vi "J1939 - Workspace Control.vi"() -> ()   [LabVIEW 2023, in "J1939 Workspace Object.lvlib"]
doc: "Sample numeric display item."
uses:
  J1939 Workspace Object.lvlib
  <vilib>/NI VeriStand/Display Template Support/DisplayTemplateSupport.llb/cluster_Screen Item Settings.ctl
  <vilib>/NI VeriStand/Display Template Support/DisplayTemplateSupport.llb/cluster_Graph Scale Settings.ctl
  <vilib>/NI VeriStand/Display Template Support/DisplayTemplateSupport.llb/cluster_Graph Plot Settings.ctl
  NationalInstruments.VeriStand.SystemStorage
  Workspace Shared/Types/UI.StateVariables.ctl
  <vilib>/NI VeriStand/Display Template Support/DisplayTemplateSupport.llb/enum_Display Template Handler Minimal To Widget Msg.ctl
  <vilib>/NI VeriStand/Execution/Workspace/SystemStateRegEventRef.ctl
  <vilib>/NI VeriStand/Execution/Workspace/Target State Info.ctl
  <vilib>/NI VeriStand/Execution/Workspace/Target State.ctl
  Workspace Shared/Types/Private Data.ctl
  <vilib>/NI/STM/TCP/TCP Connection Info.ctl
  <vilib>/NI/STM/SubVIs/MetaDataElement.ctl
  Addon/Addon Shared/Types/Error Cluster.ctl
  Addon/Addon Shared/Types/Error Types.ctl
  <vilib>/NI VeriStand/Display Template Support/DisplayTemplateSupport.llb/enum_Display Template Handler Minimal To Workspace.ctl
  <vilib>/NI VeriStand/Execution/Workspace/WorkspaceAPI.ctl
  <vilib>/NI VeriStand/Execution/Workspace/SystemStateEventRef.ctl
  Workspace Shared/Types/UI.Refs.ctl
  SubModules/CAN-Streaming-Support/Source/UIs/Workspace Shared/Types/Host Stream Queue Refs.ctl
  SubModules/CAN-Streaming-Support/Source/UIs/Workspace Shared/Types/Host Stream Queue Type.ctl
  SubModules/CAN-Streaming-Support/Source/UIs/Workspace Shared/Types/Host Stream Queue Command.ctl
  <vilib>/xnet/xnet.llb/XNET Frame CAN.ctl
  <vilib>/xnet/xnet.llb/XNET Frame Type CAN.ctl
  Addon/Support Libraries/J1939 Utilities/SubVIs/Convert CAN Arb ID to J1939 ID.vi
  <vilib>/NI VeriStand/Display Template Support/DisplayTemplateSupport.llb/sub_Display Template Handler Custom.vi
  Addon/Addon Shared/J1939 Addon Shared.lvlib
  <vilib>/NI/STM/NI STM.lvlib
  Workspace Shared/J1939 Workspace Shared.lvlib
  <vilib>/NI VeriStand/Execution/Workspace/NI_VS Workspace ExecutionAPI.lvlib
  Addon/Support Libraries/J1939 Utilities/J1939 Utilities.lvlib
  SubModules/CAN-Streaming-Support/Source/UIs/Workspace Shared/CAN Stream Support Workspace Shared.lvlib
  NationalInstruments.VeriStand.ClientAPI
panel:
  in  "Tab Control":enum32{"DTCs", "RQST", "RAW FRAME"}(tab)
  in  "Refresh Continuous":bool
  in  "Clear DTC":bool
  in  "Refresh DTCs":bool
  in  "DTCs":i32(listbox)
  in  "Addresses":string(tree)
  in  "Refresh Addresses":bool
  out "Response":string
  in  "Request":bool
  in  "PGN":u32 format="%.0x"
  in  "DA":u8(ring)
  in  "Clear Array":bool
  in  "RAW":bool
  out "Priority":u8 format="%02x"
  out "SA":u8 format="%02x"
  out "PGN":u32 format="%06x"
  in  "Identifier":u32 format="%08x"
  in  "Data":u8[](array[numeric])=[0, 0, 0, 0, 0, 0, 0, 0] format="%.0x"
  in  "Errors":bool
  out "Device":string
  in  "NIVS.Workspace Event":refnum<event-registration>
  in  "NIVS.Gateway IP Address":string
  in  "NIVS.System Definition Root":refnum<k24>
  in  "Item.Data":T1
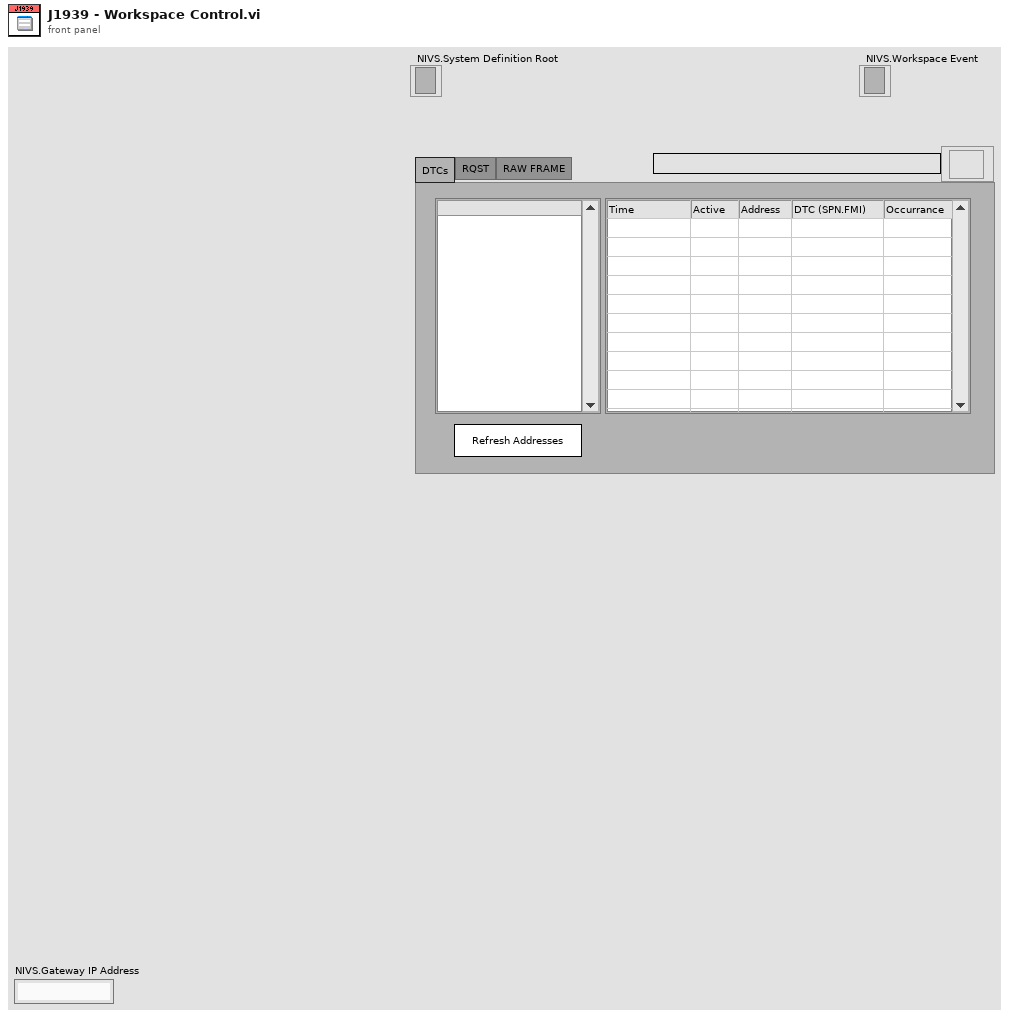
[diagram p1: front panel]
types:
  T1 = typedef "cluster_Screen Item Settings.ctl" = cluster{"Template VI":string, "Position X":i32, "Position Y":i32, "Custom":string, "Show Title Bar":bool, "ID":i32, "Always On Top":bool, "Allow Resize":bool, "Allow Minimize":bool, "Allow Close":bool, "Size to Screen":bool, "Screen.ID":i32, "State":enum16{"Normal", "New"}, "Title":string, "Window Bounds":cluster{"[0]":i16, "[1]":i16, "[2]":i16, "[3]":i16}, "Channel Ref":u64, "Unit":string, "Default Units?":bool, "Flash Limit?":bool, "Color 1":u32, "Color 2":u32, "Color 3":u32, "Color 4":u32, "Bck Color":u32, "Fore Color":u32, "Limit 1":dbl, "Limit 2":dbl, "Limit 3":dbl, "Limit 4":dbl, "Limit Mode 1":i32, "Limit Mode 2":i32, "Limit Mode 3":i32, "Limit Mode 4":i32, "Scale Precision":i32, "Scale Min":dbl, "Scale Max":dbl, "Format":i32, "Precision":i32, "Background Type":i32, "IDs":i32[], "Units":string[], "Labels":string[], "Scale Factor":dbl, "Scale Offset":dbl, "YScale Index":u32[], "XScale":T2, "YScales":T2[], "Plots":T3[], "Update Period":dbl, "History Length":dbl, "My.Ref":refnum<vi>, "Is Control?":bool, "Channel Paths":string[], "Custom Data":variant}
  T2 = typedef "cluster_Graph Scale Settings.ctl" = cluster{"Format":u8, "Precision":u8, "Fit":u8, "Label":string, "Use Default Label":bool, "Label Visible":bool, "Min":dbl, "Max":dbl}
  T3 = typedef "cluster_Graph Plot Settings.ctl" = cluster{"Bar Style":u8, "Fill To":i16, "Fill/PtColor":u32, "Line Style":u8, "Line Width":u8, "Color":u32, "Interp":u8, "Point Style":u8}
  T4 = typedef "J1939 Workspace Shared.lvlib/UI.StateVariables.ctl" = cluster{"NIVS.Gateway IP Address":string, "LaunchConfig.Ref":refnum<user-event>, "Events.Refs":cluster{"LaunchConfig":refnum<event-registration>, "SystemChange":T5, "NIVS.Workspace":refnum<event-registration>}, "State":T6, "TCP.Refs":T7, "Addresses.LUT":variant, "Errors.Q":refnum<queue>, "NIVS.SysDefRoot":refnum<k24>, "State.Notifier":refnum<user-event>, "NIVS.Workspace":T9, "DTCs.Refresh":bool, "NIVS.State.Refs":T10, "UI.Refs":T11, "Addon.Connected":bool, "DTCs.Timer":u32, "Mode.Tool?":bool, "Stream.Qs":T12, "NIVS.SysDef":path}
  T5 = typedef "NI_VS Workspace ExecutionAPI.lvlib/SystemStateRegEventRef.ctl" = refnum<event-registration>
  T6 = typedef "J1939 Workspace Shared.lvlib/Private Data.ctl" = cluster{"PGN":u32, "DA":u8, "CD Path":string, "CD IP":string}
  T7 = typedef "NI STM.lvlib/TCP Connection Info.ctl" = cluster{"connection ID":refnum<k5>, "meta data":T8[]}
  T8 = typedef "NI STM.lvlib/MetaDataElement.ctl" = string
  T9 = typedef "NI_VS Workspace ExecutionAPI.lvlib/WorkspaceAPI.ctl" = refnum<k24>
  T10 = typedef "NI_VS Workspace ExecutionAPI.lvlib/SystemStateEventRef.ctl" = cluster{"CustDatRef":refnum<user-event>, "EvtRef":refnum<k27>, "Target State User Event":refnum<user-event>}
  T11 = typedef "J1939 Workspace Shared.lvlib/UI.Refs.ctl" = cluster{"ParentVI":refnum<vi>, "DTCs":refnum<vi>, "Addresses":refnum<vi>, "Device":refnum<vi>, "Data":refnum<vi>, "Identifier":refnum<vi>, "PGN":refnum<vi>, "DA":refnum<vi>, "Refresh Continuous":refnum<vi>, "Errors":refnum<vi>, "Refresh Addresses":refnum<vi>, "Refresh DTCs":refnum<vi>, "Clear DTC":refnum<vi>, "Request":refnum<vi>, "Clear Array":refnum<vi>, "RAW":refnum<vi>, "SA":refnum<vi>, "PGN Ind":refnum<vi>, "Priority":refnum<vi>, "Response":refnum<vi>, "Reset Filter":refnum<vi>, "Enable Stream":refnum<vi>, "Log":refnum<vi>, "Clear History":refnum<vi>, "Sort By ID":refnum<vi>, "Pause":refnum<vi>, "Table Control":refnum<vi>, "Status":refnum<vi>, "Type Filter":refnum<vi>, "Filter IDs":refnum<vi>, "Host Filter":refnum<vi>, "Direction Filter":refnum<vi>, "Stream Connected":refnum<vi>}
  T12 = typedef "CAN Stream Support Workspace Shared.lvlib/Host Stream Queue Refs.ctl" = cluster{"Cmd Q":refnum<queue>, "XNET Frames":refnum<queue>}
  T13 = typedef "enum_Display Template Handler Minimal To Workspace.ctl" = cluster{"Operation":enum16{"SetCustomData", "DeleteItem"}, "Data":variant}
  T14 = typedef "enum_Display Template Handler Minimal To Widget Msg.ctl" = enum16{"Stop", "LaunchConfigDialog"}
  T15 = enum8{"Enabled", "Disabled", "Disabled and Grayed Out"}
  T16 = cluster{"LaunchConfig":refnum<event-registration>, "SystemChange":T5, "NIVS.Workspace":refnum<event-registration>}
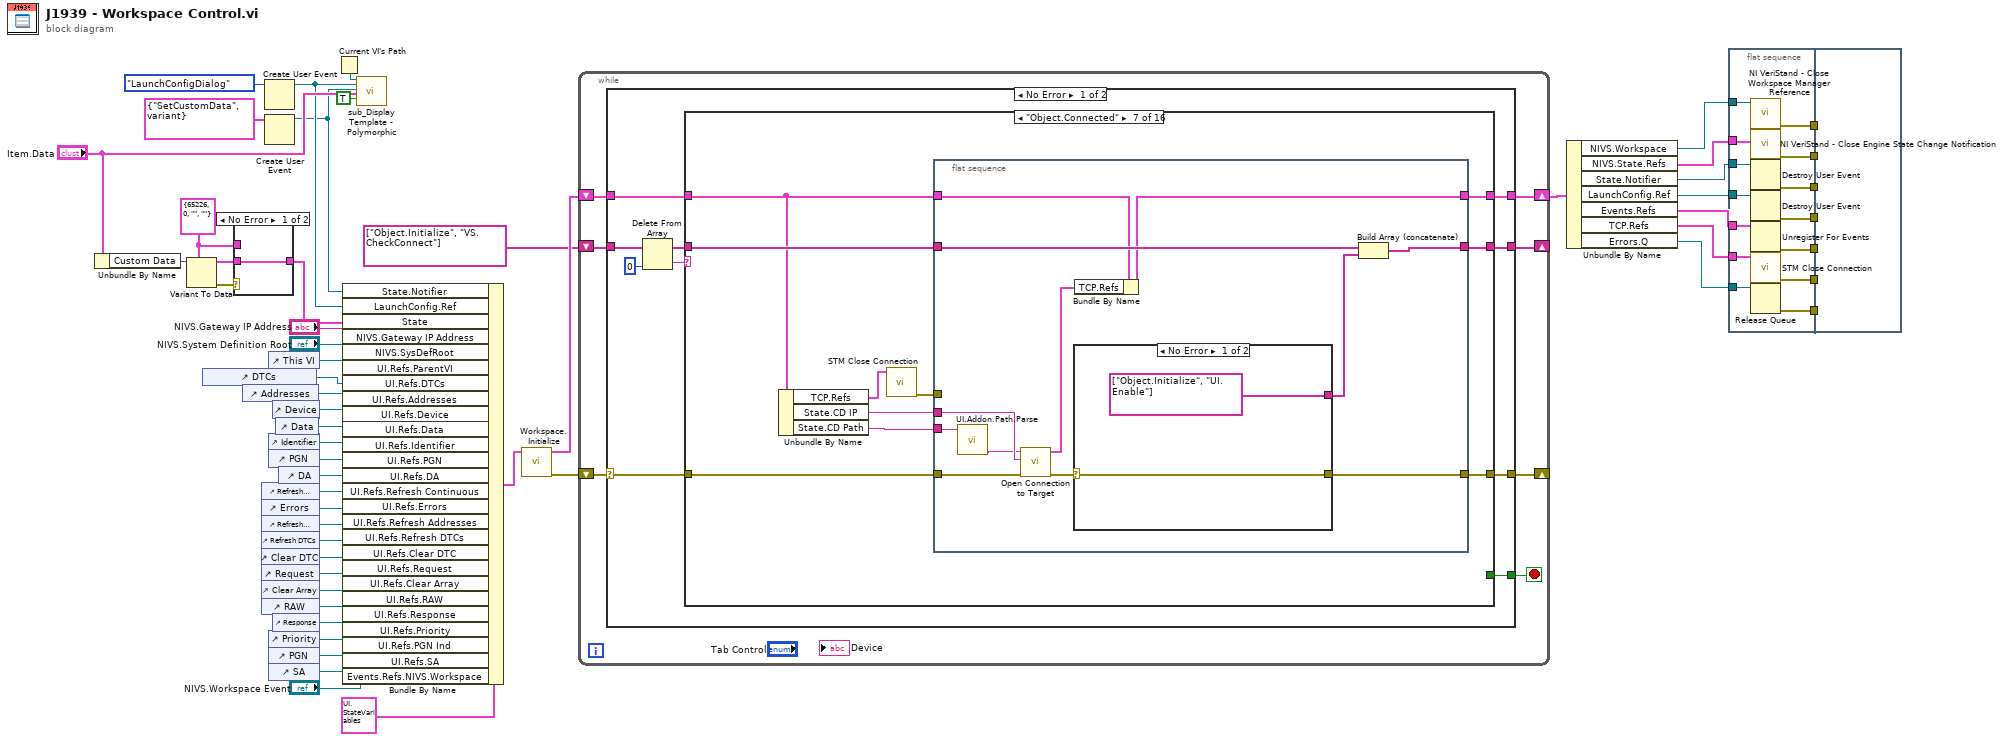
[diagram p0: block diagram]
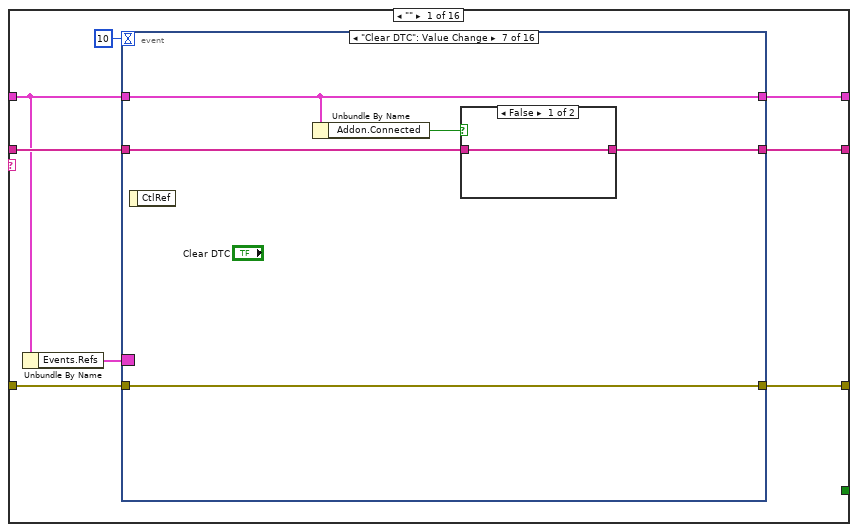
[diagram p2: hidden frame]
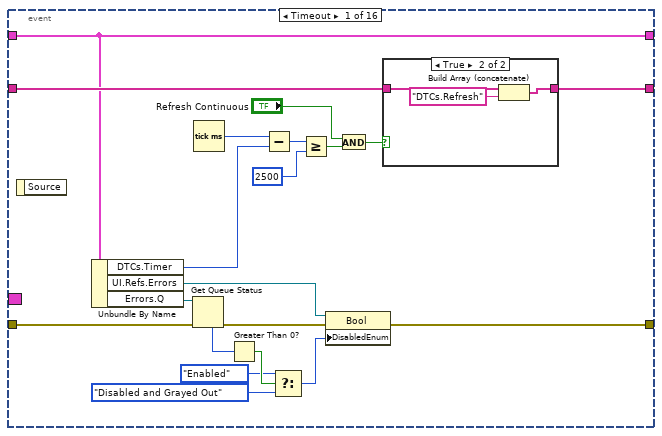
[diagram p3: hidden frame]
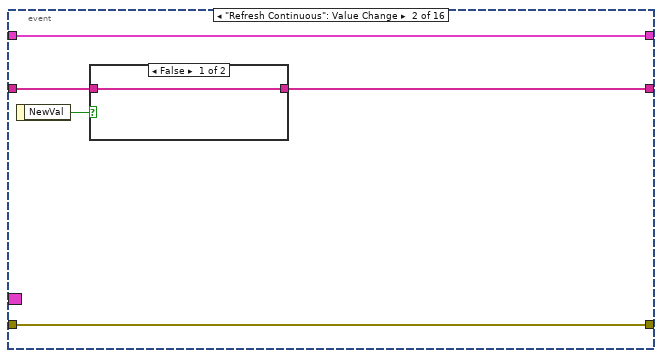
[diagram p5: hidden frame]
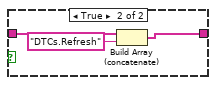
[diagram p6: hidden frame]
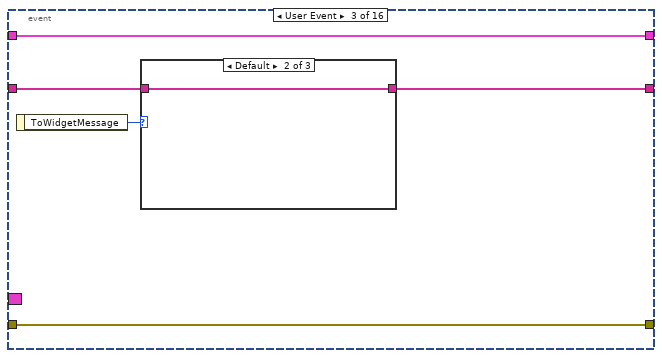
[diagram p7: hidden frame]
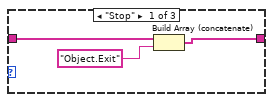
[diagram p8: hidden frame]
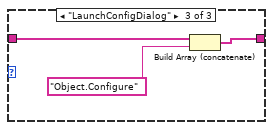
[diagram p9: hidden frame]
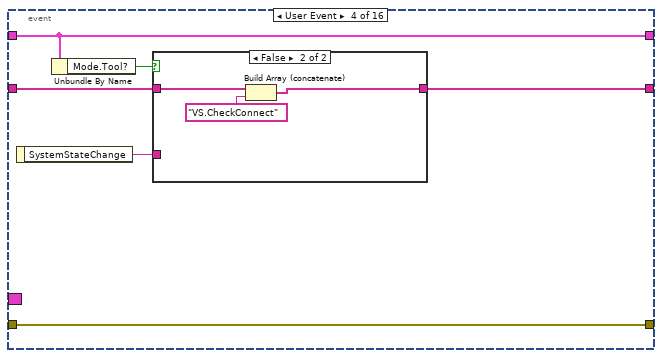
[diagram p10: hidden frame]
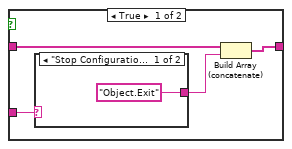
[diagram p11: hidden frame]
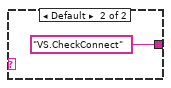
[diagram p12: hidden frame]
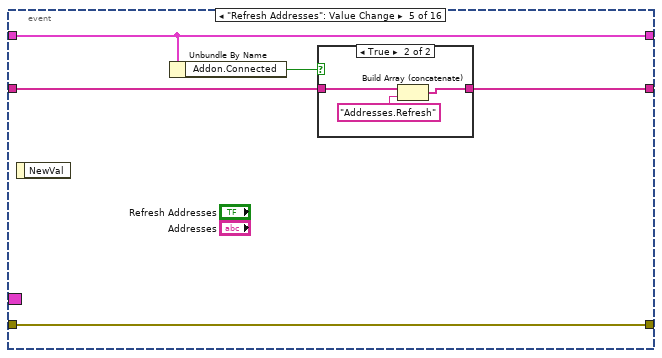
[diagram p13: hidden frame]
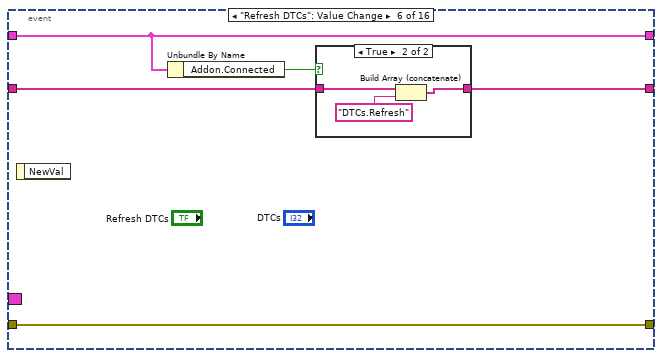
[diagram p15: hidden frame]
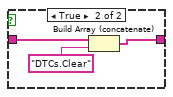
[diagram p17: hidden frame]
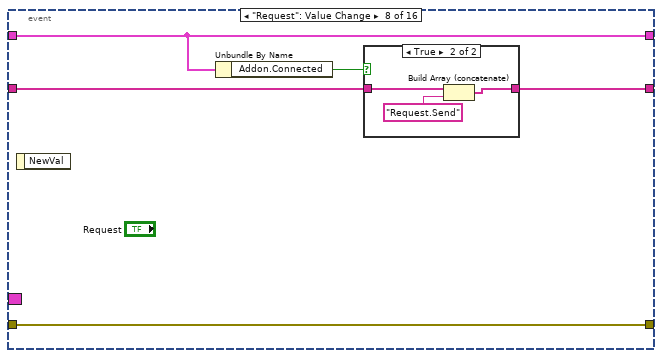
[diagram p18: hidden frame]
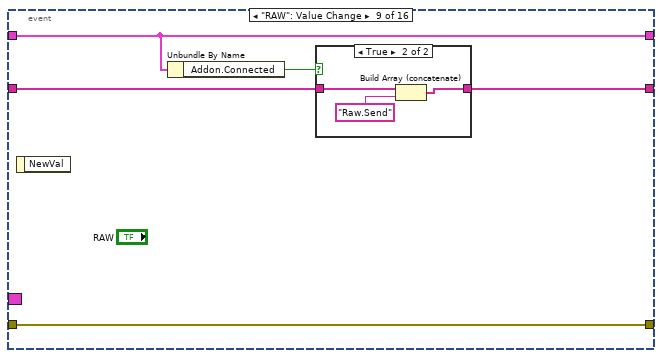
[diagram p20: hidden frame]
diagram:
  w51 = T6 {"PGN"=65226, "DA"=0, "CD Path"="", "CD IP"=""} ("Cluster")
  n1 = Unbundle By Name("Item.Data") -> ("Custom Data"=w48:variant)
  n2 = Variant To Data(type=w51, Variant=w48) -> (data=w50:T6, error out=w49:errorcluster)  [unwired: 1 in]
  n3 = control-ref of="DTCs"() -> (w35:refnum<vi>)
  n4 = case shown="No Error" w49 {
    tunnel: w50 -> [w56 _]
    tunnel: [w56 w57] -> w7
    tunnel: w51 -> [_ w57]
    frame No Error {
    }
    frame Error {
    }
  }
  n5 = control-ref of="Addresses"() -> (w34:refnum<vi>)
  n6 = control-ref of="Refresh Continuous"() -> (w28:refnum<vi>)
  n7 = control-ref of="Errors"() -> (w27:refnum<vi>)
  n8 = control-ref of="Refresh Addresses"() -> (w26:refnum<vi>)
  n9 = control-ref of="Refresh DTCs"() -> (w25:refnum<vi>)
  n10 = control-ref of="Clear DTC"() -> (w24:refnum<vi>)
  n11 = control-ref of="Request"() -> (w23:refnum<vi>)
  n12 = control-ref of="Clear Array"() -> (w22:refnum<vi>)
  n13 = control-ref of="RAW"() -> (w21:refnum<vi>)
  n14 = Create User Event(user event datatype=enum_Display_Template_Handler_Minimal_To_Widget_Msg."LaunchConfigDialog" ("ToWidgetMessage")) -> (user event=w6:refnum<user-event>)  [unwired: 1 in, 1 out]
  n15 = Create User Event(user event datatype=T13 {"Operation"=enum."SetCustomData", "Data"=variant} ("Data")) -> (user event=w5:refnum<user-event>)  [unwired: 1 in, 1 out]
  n16 = control-ref of="This VI"() -> (w36:refnum<vi>)
  n17 = control-ref of="Identifier"() -> (w31:refnum<vi>)
  n18 = control-ref of="PGN"() -> (w30:refnum<vi>)
  n19 = control-ref of="Priority"() -> (w2:refnum<vi>)
  n20 = control-ref of="PGN"() -> (w3:refnum<vi>)
  n21 = control-ref of="SA"() -> (w4:refnum<vi>)
  n22 = control-ref of="Device"() -> (w33:refnum<vi>)
  n23 = control-ref of="Response"() -> (w1:refnum<vi>)
  n24 = control-ref of="Data"() -> (w32:refnum<vi>)
  n25 = control-ref of="DA"() -> (w29:refnum<vi>)
  n26 = Current VI's Path() -> (path=w53:path)
  n27 = Bundle By Name(cluster=T4 {"NIVS.Gateway IP Address"="", "LaunchConfig.Ref"=refnum, "Events.Refs"={"LaunchConfig"=refnum, "SystemChange"=refnum, "NIVS.Workspace"=refnum}, "State"={"PGN"=0, "DA"=0, "CD Path"="", "CD IP"=""}, "TCP.Refs"={"connection ID"=refnum, "meta data"=[]}, "Addresses.LUT"=variant, "Errors.Q"=refnum, "NIVS.SysDefRoot"=refnum, "State.Notifier"=refnum, "NIVS.Workspace"=refnum, "DTCs.Refresh"=FALSE, "NIVS.State.Refs"={"CustDatRef"=refnum, "EvtRef"=refnum, "Target State User Event"=refnum}, "UI.Refs"={"ParentVI"=refnum, "DTCs"=refnum, "Addresses"=refnum, "Device"=refnum, "Data"=refnum, "Identifier"=refnum, "PGN"=refnum, "DA"=refnum, "Refresh Continuous"=refnum, "Errors"=refnum, "Refresh Addresses"=refnum, "Refresh DTCs"=refnum, "Clear DTC"=refnum, "Request"=refnum, "Clear Array"=refnum, "RAW"=refnum, "SA"=refnum, "PGN Ind"=refnum, "Priority"=refnum, "Response"=refnum, "Reset Filter"=refnum, "Enable Stream"=refnum, "Log"=refnum, "Clear History"=refnum, "Sort By ID"=refnum, "Pause"=refnum, "Table Control"=refnum, "Status"=refnum, "Type Filter"=refnum, "Filter IDs"=refnum, "Host Filter"=refnum, "Direction Filter"=refnum, "Stream Connected"=refnum}, "Addon.Connected"=FALSE, "DTCs.Timer"=0, "Mode.Tool?"=FALSE, "Stream.Qs"={"Cmd Q"=refnum, "XNET Frames"=refnum}, "NIVS.SysDef"=path ""}, "State.Notifier"=w5, "LaunchConfig.Ref"=w6, "State"=w7, "NIVS.Gateway IP Address"="NIVS.Gateway IP Address", "NIVS.SysDefRoot"="NIVS.System Definition Root", "UI.Refs.ParentVI"=w36, "UI.Refs.DTCs"=w35, "UI.Refs.Addresses"=w34, "UI.Refs.Device"=w33, "UI.Refs.Data"=w32, "UI.Refs.Identifier"=w31, "UI.Refs.PGN"=w30, "UI.Refs.DA"=w29, "UI.Refs.Refresh Continuous"=w28, "UI.Refs.Errors"=w27, "UI.Refs.Refresh Addresses"=w26, "UI.Refs.Refresh DTCs"=w25, "UI.Refs.Clear DTC"=w24, "UI.Refs.Request"=w23, "UI.Refs.Clear Array"=w22, "UI.Refs.RAW"=w21, "UI.Refs.Response"=w1, "UI.Refs.Priority"=w2, "UI.Refs.PGN Ind"=w3, "UI.Refs.SA"=w4, "Events.Refs.NIVS.Workspace"="NIVS.Workspace Event") -> (w38:T4)
  n28 = call-poly <vilib>:"sub_Display Template - Polymorphic.vi"("Parent.Path"=w53, "ToWidgetEvent"=w6, "ToWorkspace"=w5, "Item.Data"="Item.Data", "Resizable"=TRUE) -> ()  [unwired: 1 in, 14 out]
  n29 = call "Workspace.Initialize.vi"("State"=w38) -> ("error out"=w37:errorcluster, "State"=w20:T4)  [unwired: 9 in]
  n30 = while {
    shift-right: [w62] -> _
    shift-left: w37 -> [w63]
    shift-right: [w58] -> w18
    shift-left: w20 -> [w61]
    shift-right: [w59] -> _
    shift-left: string[] ["Object.Initialize", "VS.CheckConnect"] -> [w60]
    stop <- w64 stop-if-true
    n31 = case shown="No Error" w63 {
      selector: w63 -> [w65 w451]
      tunnel: [w74 FALSE] -> w64
      tunnel: [w66 w449] -> w62
      tunnel: w61 -> [w73 w446]
      tunnel: w60 -> [w71 w447]
      tunnel: [w68 w447] -> w59
      tunnel: [w67 w446] -> w58
      frame No Error {
        n32 = Delete From Array(array=w71, index=0) -> (deleted portion=w70:string, array with subset deleted=w69:string[])  [unwired: 1 in]
        n33 = case shown="\"Object.Connected\"" w70 {
          selector: w70 -> [_ _ _ _ _ _ _ _ _ _ _ _ _ _ _ w441]
          tunnel: [_ _ _ _ _ _ _ _ TRUE _ _ _ _ _ _ _] -> w74
          tunnel: w73 -> [w76 w239 w248 w265 w293 w299 w333 w361 w364 w369 w393 w401 w413 w426 w432 w444]
          tunnel: w69 -> [w80 w246 w258 w274 w295 w297 w339 w357 w365 w367 w394 w402 w409 w428 w439 w445]
          tunnel: [w81 w246 w258 w274 w295 w296 w338 w357 w365 w366 w394 w402 w409 w428 w439 w445] -> w68
          tunnel: [w79 w236 w247 w275 w293 w298 w332 w360 w364 w370 w393 w400 w410 w427 w433 w444] -> w67
          tunnel: [w78 w235 w257 w260 w292 w302 w335 w356 w363 w378 w389 w395 w408 w429 w434 w443] -> w66
          tunnel: w65 -> [w77 w235 w257 w261 w294 w303 w334 w356 w363 w379 w388 w395 w408 w430 w435 w443]
          frame "" {
            n34 = Unbundle By Name(w76) -> ("Events.Refs"=w75:T16)
            n35 = event shown="[6] \"Clear DTC\": Value Change" {
              selector: w75 -> [_ _ _ _ _ _ _ _ _ _ _ _ _ _ _ _]
              dyn-events: _ -> [_ _ _ _ _ _ _ _ _ _ _ _ _ _ _ _]
              timeout: 10 -> [_ _ _ _ _ _ _ _ _ _ _ _ _ _ _ _]
              tunnel: w76 -> [w91 w110 w120 w129 w146 w154 w161 w172 w181 w190 w199 w203 w210 w220 w225 w234]
              tunnel: [w92 w108 w116 w132 w144 w152 w162 w170 w179 w188 w198 w204 w212 w216 w222 w231] -> w81
              tunnel: w80 -> [w93 w109 w117 w133 w145 w153 w163 w171 w180 w189 w201 w204 w212 w217 w223 w232]
              tunnel: [w91 w110 w120 w129 w146 w154 w161 w172 w181 w190 w199 w203 w210 w220 w225 w234] -> w79
              tunnel: [w85 w111 w119 w130 w147 w156 w165 w174 w183 w192 w200 w202 w211 w219 w224 w233] -> w78
              tunnel: w77 -> [w87 w111 w119 w130 w147 w156 w165 w174 w183 w192 w200 w202 w211 w219 w224 w233]
              event Timeout {
                n36 = event-data() -> ()  [unwired: 2 out]
                n37 = Unbundle By Name(w91) -> ("DTCs.Timer"=w84:u32, "UI.Refs.Errors"=w89:refnum<vi>, "Errors.Q"=w90:refnum<queue>)
                n38 = Get Queue Status(queue=w90, error in (no error)=w87) -> (error out=w88:errorcluster, # elements in queue=w102:i32)  [unwired: 1 in, 6 out]
                n39 = Tick Count (ms)() -> (millisecond timer value=w96:u32)
                n40 = Greater Than 0?(x=w102) -> (x > 0?=w101:bool)
                n41 = Subtract(x=w96, y=w84) -> (x-y=w98:u32)
                n42 = Select(t=T15."Enabled" ("Disabled"), s=w101, f=T15."Disabled and Grayed Out") -> (s? t:f=w86:T15)
                n43 = Greater Or Equal?(x=w98, y=u32 2500) -> (x >= y?=w83:bool)
                n44 = property class="Bool"(reference=w89, error in=w88, "DisabledEnum"=w86) -> (error out=w85:errorcluster)  [unwired: 1 out]
                n45 = And(x="Refresh Continuous", y=w83) -> (x .and. y?=w94:bool)
                n46 = case shown="True" w94 {
                  tunnel: w93 -> [w103 w105]
                  tunnel: [w103 w104] -> w92
                  frame False {
                  }
                  frame True {
                    n47 = Build Array (concatenate)(w105, "DTCs.Refresh" ("NewVal")) -> (w104:string[])
                  }
                }
              }
              event "Refresh Continuous": Value Change {
                n48 = event-data() -> ("NewVal"=w107:bool)  [unwired: 1 out]
                n49 = case shown="False" w107 {
                  tunnel: w109 -> [w112 w114]
                  tunnel: [w112 w113] -> w108
                  frame False {
                  }
                  frame True {
                    n50 = Build Array (concatenate)(w114, "DTCs.Refresh" ("NewVal")) -> (w113:string[])
                  }
                }
              }
              event User Event {
                n51 = event-data() -> ("ToWidgetMessage"=w118:T14)  [unwired: 1 out]
                n52 = case shown="Default" w118 {
                  tunnel: w117 -> [w123 w124 w127]
                  tunnel: [w122 w124 w126] -> w116
                  frame "Stop" {
                    n53 = Build Array (concatenate)(w123, "Object.Exit") -> (w122:string[])
                  }
                  frame Default {
                  }
                  frame "LaunchConfigDialog" {
                    n54 = Build Array (concatenate)(w127, "Object.Configure") -> (w126:string[])
                  }
                }
              }
              event User Event {
                n55 = event-data() -> ("SystemStateChange"=w128:string)  [unwired: 1 out]
                n56 = Unbundle By Name(w129) -> ("Mode.Tool?"=w131:bool)
                n57 = case shown="False" w131 {
                  tunnel: w133 -> [w137 w142]
                  tunnel: [w136 w141] -> w132
                  tunnel: w128 -> [w135 _]
                  frame True {
                    # "System state not connected"
                    n58 = case shown="\"Stop Configuration\"" w135 {
                      tunnel: ["Object.Exit" "VS.CheckConnect"] -> w134
                      frame "Stop Configuration" {
                      }
                      frame Default {
                      }
                    }
                    n59 = Build Array (concatenate)(w137, w134) -> (w136:string[])
                  }
                  frame False {
                    # "System state is connected"
                    n60 = Build Array (concatenate)(w142, "VS.CheckConnect") -> (w141:string[])
                  }
                }
              }
              event "Refresh Addresses": Value Change {
                n61 = event-data() -> ()  [unwired: 2 out]
                n62 = Unbundle By Name(w146) -> ("Addon.Connected"=w143:bool)
                n63 = case shown="True" w143 {
                  tunnel: w145 -> [w148 w150]
                  tunnel: [w148 w149] -> w144
                  frame False {
                  }
                  frame True {
                    n64 = Build Array (concatenate)(w150, "Addresses.Refresh") -> (w149:string[])
                  }
                }
              }
              event "Refresh DTCs": Value Change {
                n65 = event-data() -> ()  [unwired: 2 out]
                n66 = Unbundle By Name(w154) -> ("Addon.Connected"=w155:bool)
                n67 = case shown="True" w155 {
                  tunnel: w153 -> [w157 w159]
                  tunnel: [w157 w158] -> w152
                  frame False {
                  }
                  frame True {
                    n68 = Build Array (concatenate)(w159, "DTCs.Refresh") -> (w158:string[])
                  }
                }
              }
              event "Clear DTC": Value Change {
                n69 = event-data() -> ()  [unwired: 2 out]
                n70 = Unbundle By Name(w161) -> ("Addon.Connected"=w164:bool)
                n71 = case shown="False" w164 {
                  tunnel: w163 -> [w166 w168]
                  tunnel: [w166 w167] -> w162
                  frame False {
                  }
                  frame True {
                    n72 = Build Array (concatenate)(w168, "DTCs.Clear") -> (w167:string[])
                  }
                }
              }
              event "Request": Value Change {
                n73 = event-data() -> ()  [unwired: 2 out]
                n74 = Unbundle By Name(w172) -> ("Addon.Connected"=w173:bool)
                n75 = case shown="True" w173 {
                  tunnel: w171 -> [w175 w177]
                  tunnel: [w175 w176] -> w170
                  frame False {
                  }
                  frame True {
                    n76 = Build Array (concatenate)(w177, "Request.Send") -> (w176:string[])
                  }
                }
              }
              event "RAW": Value Change {
                n77 = event-data() -> ()  [unwired: 2 out]
                n78 = Unbundle By Name(w181) -> ("Addon.Connected"=w182:bool)
                n79 = case shown="True" w182 {
                  tunnel: w180 -> [w184 w186]
                  tunnel: [w184 w185] -> w179
                  frame False {
                  }
                  frame True {
                    n80 = Build Array (concatenate)(w186, "Raw.Send") -> (w185:string[])
                  }
                }
              }
              event "Clear Array": Value Change {
                n81 = event-data() -> ()  [unwired: 2 out]
                n82 = Unbundle By Name(w190) -> ("Addon.Connected"=w191:bool)
                n83 = case shown="True" w191 {
                  tunnel: w189 -> [w193 w195]
                  tunnel: [w193 w194] -> w188
                  frame False {
                  }
                  frame True {
                    n84 = Build Array (concatenate)(w195, "Raw.Clear") -> (w194:string[])
                  }
                }
              }
              event "Addresses": Value Change {
                n85 = event-data() -> ()  [unwired: 2 out]
                n86 = Build Array (concatenate)(w201, "DTCs.Refresh" ("NewVal")) -> (w198:string[])
              }
              event "Identifier": Value Change {
                n87 = event-data() -> ("NewVal"=w205:u32)  [unwired: 1 out]
                n88 = call-poly "Common Conversions.vi"("Arb ID"=w205) -> ("Priority"=→"Priority":u8, "PGN"=→"PGN":u32, "Source Address"=→"SA":u8)  [unwired: 11 in, 1 out]
              }
              event "Errors": Value Change {
                n89 = event-data() -> ()  [unwired: 2 out]
                n90 = Unbundle By Name(w210) -> ("Errors.Q"=w209:refnum<queue>)
                n91 = flat-sequence {
                  tunnel: [w214] -> w213
                  tunnel: w209 -> [w214]
                  frame #0 {
                  }
                }
                n92 = call "Error Display.vi"("queue out"=w213) -> ()  [unwired: 11 in]
              }
              event Panel Close? {
                n93 = event-data() -> ()  [unwired: 5 out]
                n94 = Build Array (concatenate)(w217, "Object.Exit") -> (w216:string[])
                n95 = event-data("Discard?"=TRUE) -> ()  [unwired: 1 in, 1 out]
              }
              event User Event {
                n96 = event-data() -> ("Workspace Event"=w221:string)  [unwired: 1 out]
                n97 = case shown="\"Disconnect\", \"Shut Down\"" w221 {
                  tunnel: w223 -> [w226 w229]
                  tunnel: [w226 w228] -> w222
                  frame Default {
                  }
                  frame "Disconnect", "Shut Down" {
                    n98 = Build Array (concatenate)(w229, "Object.Exit") -> (w228:string[])
                  }
                }
              }
              event Menu Selection (User) {
                n99 = event-data() -> ("ItemTag"=w230:string)  [unwired: 1 out]
                n100 = Build Array (concatenate)(w232, w230) -> (w231:string[])
              }
            }
          }
          frame "Addresses.Refresh" {
            n101 = Unbundle By Name(w239) -> ("UI.Refs.Addresses"=w245:refnum<vi>, "UI.Refs.DA"=w244:refnum<vi>, "TCP.Refs"=w243:T7, "State"=w242:T6, "Errors.Q"=w241:refnum<queue>, "UI.Refs.ParentVI"=w240:refnum<vi>)
            n102 = call "Request Addresses Event.vi"("connection info"=w243, "DA"=w244, "Addresses"=w245, "State Variables"=w242, "Error Q"=w241, "VI Ref"=w240) -> ("connection info"=w238:T7, "Address Lookup Table Out"=w237:variant)  [unwired: 8 in]
            n103 = Bundle By Name(cluster=w239, "TCP.Refs"=w238, "Addresses.LUT"=w237) -> (w236:T4)
          }
          frame "DTCs.Clear" {
            n104 = Unbundle By Name(w248) -> ("UI.Refs.Addresses"=w251:refnum<vi>, "TCP.Refs"=w256:T7, "State"=w255:T6, "Addresses.LUT"=w254:variant, "Errors.Q"=w253:refnum<queue>, "UI.Refs.ParentVI"=w252:refnum<vi>)
            n105 = call "Clear DTCs Event.vi"("connection info"=w256, "Addresses"=w251, "State Variables"=w255, "Address Lookup Table"=w254, "Error Q"=w253, "VI Ref"=w252) -> ("connection info"=w250:T7, "Address Lookup Table Out"=w249:variant)  [unwired: 8 in]
            n106 = Bundle By Name(cluster=w248, "TCP.Refs"=w250, "Addresses.LUT"=w249) -> (w247:T4)
          }
          frame "DTCs.Refresh" {
            n107 = Unbundle By Name(w265) -> ("UI.Refs.DTCs"=w272:refnum<vi>, "UI.Refs.Addresses"=w271:refnum<vi>, "TCP.Refs"=w270:T7, "State"=w269:T6, "Addresses.LUT"=w268:variant, "Errors.Q"=w267:refnum<queue>, "UI.Refs.ParentVI"=w266:refnum<vi>, "UI.Refs.Refresh Continuous"=w262:refnum<vi>)
            n108 = property class="Bool (strict)"(reference=w262, error in=w261) -> (error out=w260:errorcluster, "Value"=w259:bool)  [unwired: 1 out]
            n109 = Not(x=w259) -> (.not. x?=w273:bool)
            n110 = flat-sequence {
              tunnel: w268 -> [w288]
              tunnel: w270 -> [w286]
              tunnel: w269 -> [w284]
              tunnel: w273 -> [w283]
              tunnel: [w287] -> w278
              tunnel: [w285] -> w277
              tunnel: w272 -> [w282]
              tunnel: w271 -> [w281]
              tunnel: w267 -> [w280]
              tunnel: w266 -> [w279]
              tunnel: [w290] -> w263
              tunnel: [w291] -> w264
              tunnel: w278 -> [w291]
              tunnel: w277 -> [w290]
              tunnel: [w289] -> w276
              frame #0 {
                n111 = call "Refresh DTCs Event.vi"("connection info"=w286, "Addresses"=w281, "DTCs"=w282, "State Variables"=w284, "Address Lookup Table"=w288, "To Top (T)"=w283, "Error Q"=w280, "VI Ref"=w279) -> ("connection info"=w285:T7, "Address Lookup Table Out"=w287:variant)  [unwired: 6 in]
              }
              frame #1 {
                n112 = Tick Count (ms)() -> (millisecond timer value=w289:u32)
              }
            }
            n113 = Bundle By Name(cluster=w265, "DTCs.Timer"=w276, "TCP.Refs"=w263, "Addresses.LUT"=w264) -> (w275:T4)
          }
          frame "Object.Initialize" {
            n114 = call "Initialize Workspace Object.vi"("error in (no error)"=w294, "State"=w293) -> ("error out"=w292:errorcluster)  [unwired: 9 in]
          }
          frame "Object.Configure" {
            n115 = Unbundle By Name(w299) -> ("State"=w301:T6, "State.Notifier"=w304:refnum<user-event>, "NIVS.SysDefRoot"=w305:refnum<k24>, "State.CD Path"=w308:string)
            n116 = call "Select Custom Device.vi"("CD Path"=w308, "NIVS.System Definition Root"=w305) -> ("Cancelled?"=w306:bool, "IP Address"=w309:string, "Custom Device Path Out"=w307:string)  [unwired: 7 in]
            n117 = case shown="False" w306 {
              tunnel: w304 -> [w311 _]
              tunnel: w309 -> [w317 _]
              tunnel: w307 -> [w318 _]
              tunnel: w303 -> [w315 w329]
              tunnel: [w315 w329] -> w302
              tunnel: w301 -> [w316 w328]
              tunnel: [w310 w328] -> w300
              tunnel: w297 -> [w314 w327]
              tunnel: [w312 w327] -> w296
              frame False {
                n118 = flat-sequence {
                  tunnel: w318 -> [w326]
                  tunnel: w317 -> [w325]
                  tunnel: w316 -> [w324]
                  tunnel: w311 -> [w321]
                  tunnel: [w320] -> w310
                  tunnel: [w319] -> _
                  frame #0 {
                    n119 = Bundle By Name(cluster=w324, "CD Path"=w326, "CD IP"=w325) -> (w320:T6)
                    n120 = Bundle By Name(cluster=T13 {"Operation"=enum."SetCustomData", "Data"=variant} ("event data"), "Data"=w320) -> (w322:T13)
                    n121 = Generate User Event(user event=w321, event data cluster=w322) -> (error out=w319:errorcluster)  [unwired: 2 in, 1 out]
                  }
                }
                n122 = Build Array (concatenate)(w314, "VS.CheckConnect") -> (w312:string[])
              }
              frame True {
              }
            }
            n123 = Bundle By Name(cluster=w299, "State"=w300) -> (w298:T4)
          }
          frame "Object.Connected" {
            n124 = Unbundle By Name(w333) -> ("TCP.Refs"=w331:T7, "State.CD IP"=w336:string, "State.CD Path"=w337:string)
            n125 = call "STM Close Connection.vi"("connection info"=w331) -> ("error out"=w330:errorcluster)  [unwired: 10 in]
            n126 = flat-sequence {
              tunnel: w339 -> [w351]
              tunnel: [w349] -> w338
              tunnel: w337 -> [w341]
              tunnel: w336 -> [w348]
              tunnel: [w346] -> w335
              tunnel: w334 -> [w345]
              tunnel: w333 -> [w343]
              tunnel: [w342] -> w332
              tunnel: w330 -> [_]
              frame #0 {
                n127 = call "UI.Addon.Path.Parse.vi"("Cached Addon Path"=w341) -> ("Addon Name"=w340:string)  [unwired: 6 in, 4 out]
                n128 = call "Open Connection to Target.vi"("error in (no error)"=w345, "IP Address"=w348, "TCP Service"=w340) -> ("error out"=w347:errorcluster, "connection info"=w344:T7)  [unwired: 7 in]
                n129 = case shown="No Error" w347 {
                  selector: w347 -> [w353 w355]
                  tunnel: [string[] ["Object.Initialize", "UI.Enable"] ("element") string[] ["Object.Initialize", "UI.Disable"] ("element")] -> w350
                  tunnel: [w353 w355] -> w346
                  frame No Error {
                  }
                  frame Error {
                  }
                }
                n130 = Bundle By Name(cluster=w343, "TCP.Refs"=w344) -> (w342:T4)
                n131 = Build Array (concatenate)(w351, w350) -> (w349:string[])
              }
            }
          }
          frame "Object.Disconnected" {
            n132 = Unbundle By Name(w361) -> ("TCP.Refs"=w359:T7)
            n133 = Bundle By Name(cluster=w361, "TCP.Refs"=T7 {"connection ID"=refnum, "meta data"=[]}) -> (w360:T4)
            n134 = call "STM Close Connection.vi"("connection info"=w359) -> ()  [unwired: 10 in, 1 out]
          }
          frame "Object.Exit" {
          }
          frame "VS.CheckConnect" {
            n135 = Unbundle By Name(w369) -> ("UI.Refs.Device"=w376:refnum<vi>, "NIVS.Workspace"=w374:T9, "NIVS.SysDefRoot"=w375:refnum<k24>, "State.CD Path"=w373:string)
            n136 = Current VI's Menubar() -> (w377:refnum<k9>)
            n137 = call "UI.Connection.State.Get.vi"("Menu Ref"=w377, "Name Ref"=w376, "error in (no error)"=w379, "Addon Path in"=w373, "NIVS.System Definition Root in"=w375, "NIVS.Workspace Ref in"=w374) -> ("error out"=w378:errorcluster, "Addon Connected?"=w368:bool, "NIVS.System Definition Root out"=w371:refnum<k24>, "NIVS.Workspace Ref out"=w372:T9)  [unwired: 1 in, 1 out]
            n138 = case shown="False" w368 {
              tunnel: w367 -> [w382 w385]
              tunnel: [w381 w384] -> w366
              frame False {
                n139 = Build Array (concatenate)(w382, string[] ["Object.Disconnected", "Object.Initialize", "UI.Disable"]) -> (w381:string[])
              }
              frame True {
                n140 = Build Array (concatenate)(w385, "Object.Connected") -> (w384:string[])
              }
            }
            n141 = Bundle By Name(cluster=w369, "NIVS.Workspace"=w372, "NIVS.SysDefRoot"=w371, "Addon.Connected"=w368) -> (w370:T4)
          }
          frame "Raw.Clear" {
            n142 = Unbundle By Name(w393) -> ("UI.Refs.Identifier"=w391:refnum<vi>, "UI.Refs.Data"=w392:refnum<vi>)
            n143 = property class="Arr (strict)"(reference=w392, error in=w388, "Value"=u8[] []) -> (error out=w390:errorcluster)  [unwired: 1 out]
            n144 = property class="DigNum (strict)"(reference=w391, error in=w390, "Val(Sgnl)"=u32 0 ("Value (Signaling)")) -> (error out=w389:errorcluster)  [unwired: 1 out]
          }
          frame "Raw.Send" {
            n145 = Unbundle By Name(w401) -> ("TCP.Refs"=w405:T7, "State"=w404:T6, "Addresses.LUT"=w403:variant, "Errors.Q"=w399:refnum<queue>, "UI.Refs.ParentVI"=w398:refnum<vi>)
            n146 = call "RAW Event.vi"("connection info"=w405, "State Variables"=w404, "Address Lookup Table"=w403, "Identifier"="Identifier", "Data"="Data", "Error Q"=w399, "VI Ref"=w398) -> ("connection info"=w397:T7, "Address Lookup Table Out"=w396:variant)  [unwired: 7 in]
            n147 = Bundle By Name(cluster=w401, "TCP.Refs"=w397, "Addresses.LUT"=w396) -> (w400:T4)
          }
          frame "Request.Send" {
            n148 = Unbundle By Name(w413) -> ("TCP.Refs"=w418:T7, "State"=w417:T6, "Addresses.LUT"=w416:variant, "Errors.Q"=w415:refnum<queue>, "UI.Refs.ParentVI"=w414:refnum<vi>)
            n149 = call "Request Event.vi"("connection info"=w418, "State Variables"=w417, "Address Lookup Table"=w416, "PGN"="PGN", "DA"="DA", "Error Q"=w415, "VI Ref"=w414) -> ("connection info"=w412:T7, "Response"=→"Response":string, "Address Lookup Table Out"=w411:variant)  [unwired: 6 in]
            n150 = Bundle By Name(cluster=w413, "TCP.Refs"=w412, "Addresses.LUT"=w411) -> (w410:T4)
          }
          frame "UI.Disable" {
            n151 = Unbundle By Name(w426) -> ("Mode.Tool?"=w422:bool, "UI.Refs"=w425:T11)
            n152 = call "Workspace.UI.DisableState.Set.vi"("Mode.Tool?"=w422, "error in (no error)"=w430, "Enable?"=FALSE, "UI.Refs"=w425) -> ("error out"=w429:errorcluster, "UI.Refs out"=w424:T11)  [unwired: 6 in]
            n153 = Bundle By Name(cluster=w426, "UI.Refs"=w424) -> (w427:T4)
          }
          frame "UI.Enable" {
            n154 = Unbundle By Name(w432) -> ("Mode.Tool?"=w431:bool, "UI.Refs"=w438:T11)
            n155 = call "Workspace.UI.DisableState.Set.vi"("Mode.Tool?"=w431, "error in (no error)"=w435, "Enable?"=TRUE, "UI.Refs"=w438) -> ("error out"=w434:errorcluster, "UI.Refs out"=w437:T11)  [unwired: 6 in]
            n156 = Bundle By Name(cluster=w432, "UI.Refs"=w437) -> (w433:T4)
          }
          frame Default {
            n157 = Concatenate Strings(w441, " is not a valid command." ("string")) -> (w440:string)
            n158 = One Button Dialog(message=w440) -> ()  [unwired: 1 in, 1 out]
          }
        }
      }
      frame Error {
        n159 = call <vilib>:"Simple Error Handler.vi"("error in (no error)"=w451) -> ("error out"=w450:errorcluster)  [unwired: 4 in, 4 out]
        n160 = call <vilib>:"Clear Errors.vi"("error in (no error)"=w450) -> ("error out"=w449:errorcluster)  [unwired: 5 in, 1 out]
      }
    }
  }
  n161 = Unbundle By Name(w18) -> ("NIVS.Workspace"=w13:T9, "NIVS.State.Refs"=w14:T10, "State.Notifier"=w16:refnum<user-event>, "LaunchConfig.Ref"=w17:refnum<user-event>, "Events.Refs"=w15:T16, "TCP.Refs"=w12:T7, "Errors.Q"=w11:refnum<queue>)
  n162 = flat-sequence {
    tunnel: w17 -> [w465]
    tunnel: w16 -> [w464]
    tunnel: w15 -> [w463]
    tunnel: w14 -> [w462]
    tunnel: w13 -> [w461]
    tunnel: w12 -> [w455]
    tunnel: w11 -> [w452]
    tunnel: [w460] -> w46
    tunnel: [w459] -> w45
    tunnel: [w458] -> w44
    tunnel: [w457] -> w43
    tunnel: [w456] -> w42
    tunnel: [w454] -> w41
    tunnel: [w453] -> w40
    tunnel: w46 -> [_]
    tunnel: w45 -> [_]
    tunnel: w44 -> [_]
    tunnel: w43 -> [_]
    tunnel: w42 -> [_]
    tunnel: w41 -> [_]
    tunnel: w40 -> [_]
    frame #0 {
      n163 = call <vilib>:"NI VeriStand - Close Workspace Manager Reference.vi"("WorkspaceManager"=w461) -> ("error out"=w460:errorcluster)  [unwired: 10 in]
      n164 = call <vilib>:"NI VeriStand - Close Engine State Change Notification.vi"("SystemStateRefs"=w462) -> ("error out"=w459:errorcluster)  [unwired: 10 in]
      n165 = Destroy User Event(user event=w464) -> (error out=w458:errorcluster)  [unwired: 1 in]
      n166 = Destroy User Event(user event=w465) -> (error out=w457:errorcluster)  [unwired: 1 in]
      n167 = Unregister For Events(event registration refnum=w463) -> (error out=w456:errorcluster)  [unwired: 1 in]
      n168 = call "STM Close Connection.vi"("connection info"=w455) -> ("error out"=w454:errorcluster)  [unwired: 10 in]
      n169 = Release Queue(queue=w452) -> (error out=w453:errorcluster)  [unwired: 2 in, 2 out]
    }
    frame #1 {
    }
  }
